vi "PrepareRollToPassReceiverRole.vi"(6 "Tactic index in":i32, 7 "first call":bool, 8 "error in (no error)":errorcluster, 10 "Game in":refnum<class "Game.lvclass">, 11 "PrepareRollToPassReceiverRole in":refnum<class "PrepareRollToPassReceiverRole.lvclass">) -> (0 "error out":errorcluster, 1 "tactic index":i32, 2 "Robot out":refnum<class "Robot.lvclass">, 3 "PrepareRollToPassReceiverRole out":refnum<class "PrepareRollToPassReceiverRole.lvclass">)   [LabVIEW 2021, in "PrepareRollToPassReceiverRole.lvclass"]
uses:
  PrepareRollToPassReceiverRole.lvclass
  Robot_class/Robot.lvclass
  Game_class/Game.lvclass
  D:/RoboIme/horie/SSL_AI/Role_class/Role.lvclass
  Utilities_class/Utilities.lvclass
  Role_class/Role.lvclass/Role.ctl
  PrepareRollToPassReceiverRole.lvclass/PrepareRollToPassReceiverRole.ctl
  AttackerStopTactic_class/States.ctl
  Tacticbook_class/Tacticbook.lvclass/Tacticbook.ctl
  AttackerStopTactic_class/AttackerStopTactic.lvclass/AttackerStopTactic.ctl
  PrepareRollToPassReceiverGoToTactic_class/PrepareRollToPassReceiverGoToTactic.lvclass/PrepareRollToPassReceiverGoToTactic.ctl
  Tacticbook_class/Read AttackerStopTactic.vi
  AttackerStopTactic_class/Read States.vi
  Tacticbook_class/Write AttackerStopTactic.vi
  Tacticbook_class/Read PrepareRollToPassReceiverGoToTactic.vi
  PrepareRollToPassReceiverGoToTactic_class/Read States.vi
  Tacticbook_class/Write PrepareRollToPassReceiverGoToTactic.vi
  Role_class/Read Tacticbook.vi
  Read number_of_tactics.vi
  Role_class/Write Tacticbook.vi
  Role_class/Write tactic_index.vi
  Role_class/Read RobotRef.vi
  Tacticbook_class/Tacticbook.lvclass
  AttackerStopTactic_class/AttackerStopTactic.lvclass
  PrepareRollToPassReceiverGoToTactic_class/PrepareRollToPassReceiverGoToTactic.lvclass
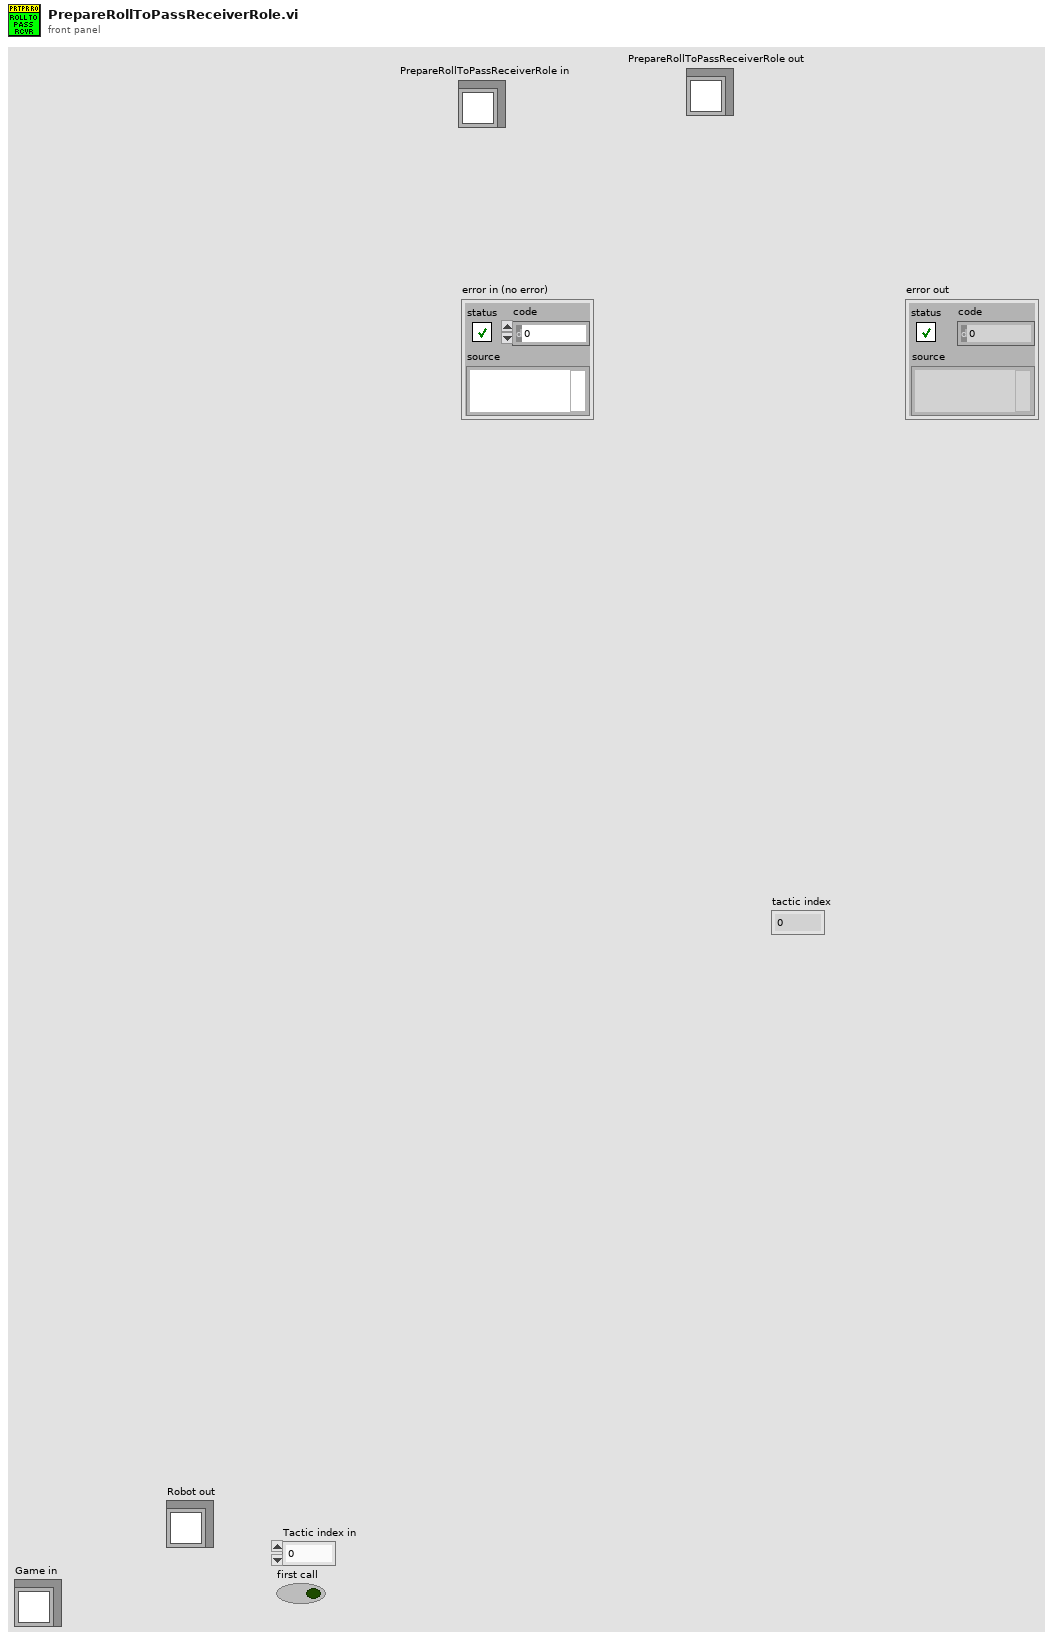
[diagram p1: front panel]
types:
  T1 = typedef "AttackerStopTactic.lvclass/States.ctl" = enum16{"Block", "AimGoal", "Exit"}
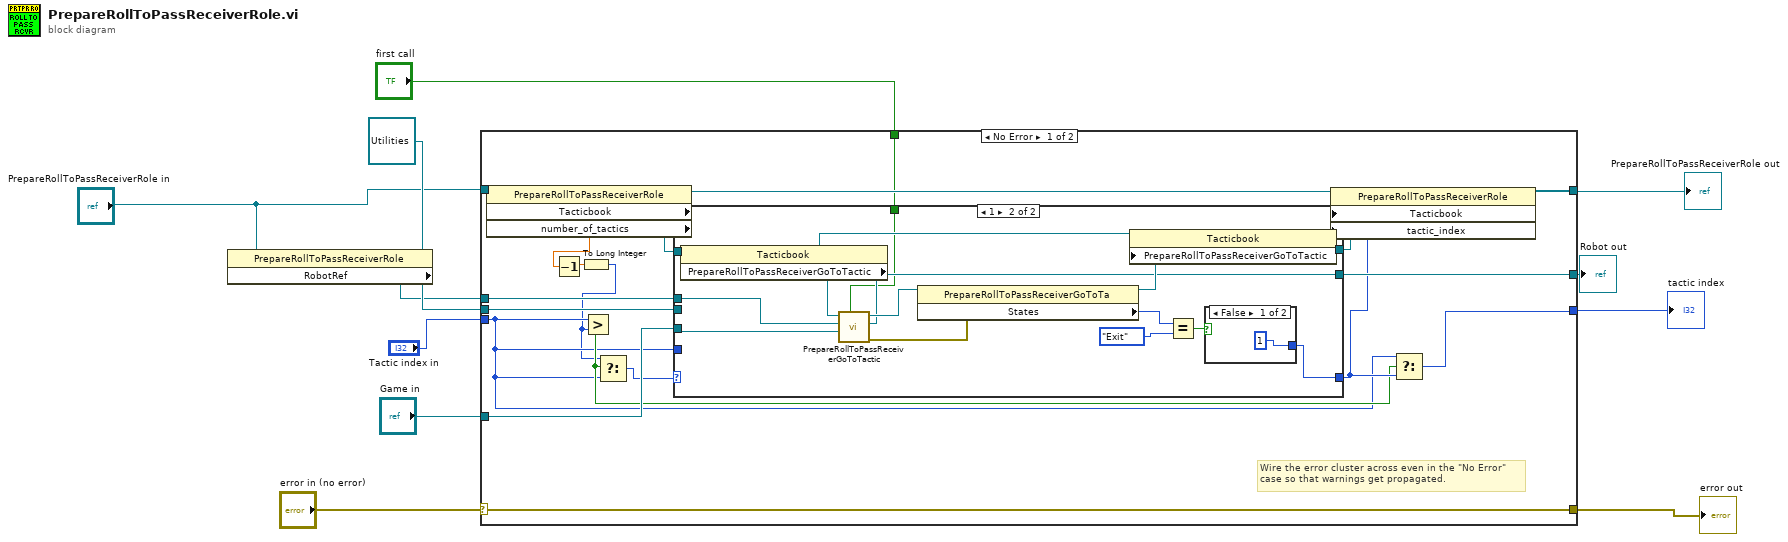
[diagram p0: block diagram]
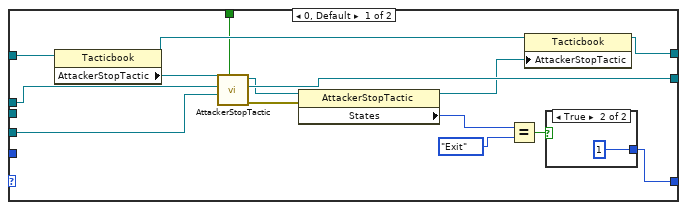
[diagram p2: hidden frame]
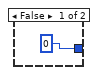
[diagram p3: hidden frame]
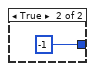
[diagram p4: hidden frame]
diagram:
  n1 = property class="PrepareRollToPassReceiverRole"(reference="PrepareRollToPassReceiverRole in") -> ("RobotRef"=w4:refnum<class "Robot.lvclass">)  [unwired: 1 in, 2 out]
  n2 = case shown="No Error" "error in (no error)" {
    selector: "error in (no error)" -> [w30 w67]
    tunnel: [w30 w67] -> w8
    tunnel: [w28 w66] -> w1
    tunnel: "PrepareRollToPassReceiverRole in" -> [w29 w66]
    tunnel: w4 -> [w25 w65]
    tunnel: [w24 w65] -> w11
    tunnel: "Game in" -> [w22 _]
    tunnel: [w17 _] -> w7
    tunnel: "Tactic index in" -> [w16 _]
    tunnel: refnum<class "Utilities.lvclass"> refnum ("Utilities in") -> [w15 _]
    tunnel: "first call" -> [w14 _]
    frame No Error {
      # "Wire the error cluster across even in the \"No Error\"\ncase so that warnings get propagated."
      n3 = property class="PrepareRollToPassReceiverRole"(reference=w29) -> (reference out=w27:refnum<class "PrepareRollToPassReceiverRole.lvclass">, "Tacticbook"=w26:refnum<class "Tacticbook.lvclass">, "number_of_tactics"=w21:dbl)  [unwired: 1 in, 1 out]
      n4 = Decrement(x=w21) -> (x-1=w12:dbl)
      n5 = To Long Integer(number=w12) -> (32bit integer=w13:i32)
      n6 = Greater?(x=w16, y=w13) -> (0:w18:bool)
      n7 = Select(t=w13, s=w18, f=w16) -> (s? t:f=w20:i32)
      n8 = case shown="1" w20 {
        tunnel: [w33 w50] -> w19
        tunnel: w26 -> [w45 w58]
        tunnel: w25 -> [w36 w53]
        tunnel: [w44 w55] -> w24
        tunnel: [w40 w54] -> w23
        tunnel: w22 -> [w37 w52]
        tunnel: w16 -> [_ _]
        tunnel: w15 -> [_ _]
        tunnel: w14 -> [w32 w48]
        frame 0, Default {
          n9 = property class="Tacticbook"(reference=w45) -> (reference out=w42:refnum<class "Tacticbook.lvclass">, "AttackerStopTactic"=w39:refnum<class "AttackerStopTactic.lvclass">)  [unwired: 1 in, 1 out]
          n10 = call-dynamic "AttackerStopTactic.vi"("first call"=w32, "Game in"=w37, "Robot"=w36, "AttackerStopTactic in"=w39) -> ("error out"=w43:errorcluster, "Robot out"=w44:refnum<class "Robot.lvclass">, "AttackerStopTactic out"=w38:refnum<class "AttackerStopTactic.lvclass">)  [unwired: 5 in]
          n11 = property class="AttackerStopTactic"(reference=w38, error in=w43) -> (reference out=w41:refnum<class "AttackerStopTactic.lvclass">, "States"=w34:T1)  [unwired: 1 out]
          n12 = Equal?(x=w34, y=States."Exit") -> (x = y?=w35:bool)
          n13 = property class="Tacticbook"(reference=w42, "AttackerStopTactic"=w41) -> (reference out=w40:refnum<class "Tacticbook.lvclass">)  [unwired: 1 in, 1 out]
          n14 = case shown="True" w35 {
            tunnel: [0 1] -> w33
            frame False {
            }
            frame True {
            }
          }
        }
        frame 1 {
          n15 = property class="Tacticbook"(reference=w58) -> (reference out=w62:refnum<class "Tacticbook.lvclass">, "PrepareRollToPassReceiverGoToTactic"=w57:refnum<class "PrepareRollToPassReceiverGoToTactic.lvclass">)  [unwired: 1 in, 1 out]
          n16 = call "PrepareRollToPassReceiverGoToTactic.vi"("first call"=w48, "Game in"=w52, "Robot"=w53, "PrepareRollToPassReceiverGoToTactic in"=w57) -> ("error out"=w51:errorcluster, "Robot out"=w55:refnum<class "Robot.lvclass">, "PrepareRollToPassReceiverGoToTactic out"=w56:refnum<class "PrepareRollToPassReceiverGoToTactic.lvclass">)  [unwired: 5 in]
          n17 = property class="PrepareRollToPassReceiverGoToTa"(reference=w56, error in=w51) -> (reference out=w61:refnum<class "PrepareRollToPassReceiverGoToTactic.lvclass">, "States"=w59:enum16{"Exit", "GoTo"})  [unwired: 1 out]
          n18 = property class="Tacticbook"(reference=w62, "PrepareRollToPassReceiverGoToTactic"=w61) -> (reference out=w54:refnum<class "Tacticbook.lvclass">)  [unwired: 1 in, 1 out]
          n19 = Equal?(x=w59, y=enum16{"Exit", "GoTo"}."Exit") -> (x = y?=w60:bool)
          n20 = case shown="False" w60 {
            tunnel: [1 -1] -> w50
            frame False {
            }
            frame True {
            }
          }
        }
      }
      n21 = property class="PrepareRollToPassReceiverRole"(reference=w27, "Tacticbook"=w23, "tactic_index"=w19) -> (reference out=w28:refnum<class "PrepareRollToPassReceiverRole.lvclass">)  [unwired: 1 in, 1 out]
      n22 = Select(t=w16, s=w18, f=w19) -> (s? t:f=w17:i32)
    }
    frame Error {
    }
  }
  "error out" <- w8
  "Robot out" <- w11
  "tactic index" <- w7
  "PrepareRollToPassReceiverRole out" <- w1
